vi "Separa_ID_list.vi"(3 "All ID list":u32[](array[numeric]) format="%x") -> (0 "Chip ID list":u32[](array[numeric]) format="%x", 1 "Layer ID list (ordered)":u32[](array[numeric]) format="%x")   [LabVIEW 2015, in "VIPM2.lvlib"]
uses:
  VIPM2.lvlib
panel:
  # "Separa: ID de layer, ID de chip"
  # "Ordena les llistes de sortida"
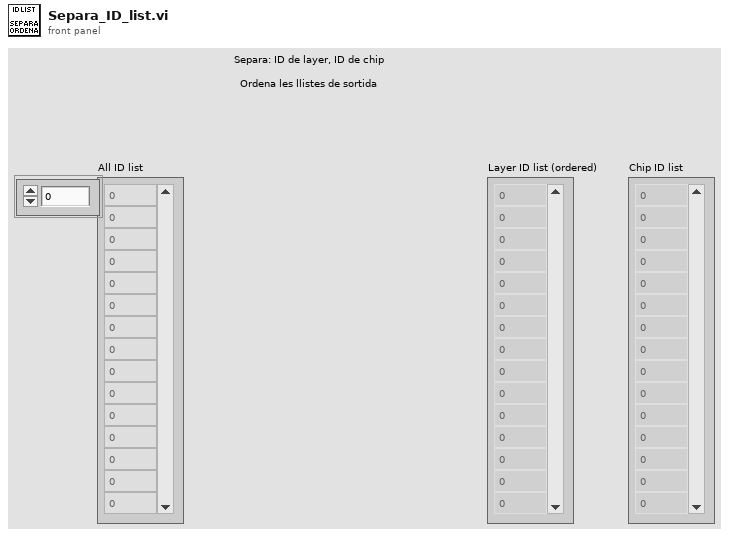
[diagram p1: front panel]
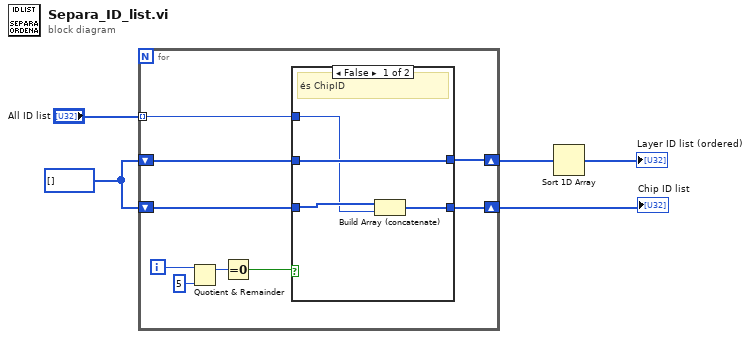
[diagram p0: block diagram]
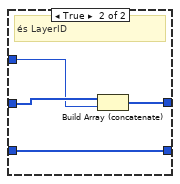
[diagram p2: hidden frame]
diagram:
  w4 = u32[] []
  n1 = for {
    tunnel: "All ID list" -> [w10] mode=indexing
    shift-right: [w9] -> w3
    shift-left: w4 -> [w8]
    shift-right: [w6] -> w1
    shift-left: w4 -> [w7]
    i -> [w14]
    n2 = Quotient & Remainder(x=w14, y=5) -> (x-y*floor(x/y)=w12:i32)  [unwired: 1 out]
    n3 = Equal To 0?(x=w12) -> (x = 0?=w11:bool)
    n4 = case shown="False" w11 {
      tunnel: w10 -> [w15 w20]
      tunnel: [w18 w22] -> w9
      tunnel: w8 -> [w18 w21]
      tunnel: w7 -> [w16 w19]
      tunnel: [w17 w19] -> w6
      frame False {
        # "és ChipID"
        n5 = Build Array (concatenate) "Build Array"(w16, w15) -> (w17:u32[])
      }
      frame True {
        # "és LayerID"
        n6 = Build Array (concatenate) "Build Array"(w21, w20) -> (w22:u32[])
      }
    }
  }
  "Chip ID list" <- w1
  n7 = Sort 1D Array(array=w3) -> (sorted array=→"Layer ID list (ordered)":u32[])
